vi "디버깅실습(해당 조건부터 하이라이트).vi"() -> ()   [LabVIEW 2020]
panel:
  out "에러 출력":errorcluster
  out "불리언":bool
  out "숫자형":i32
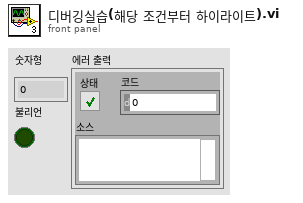
[diagram p1: front panel]
types:
  T1 = enum16{"open", "replace", "create", "open or create", "replace or create", "replace or create with confirmation"}
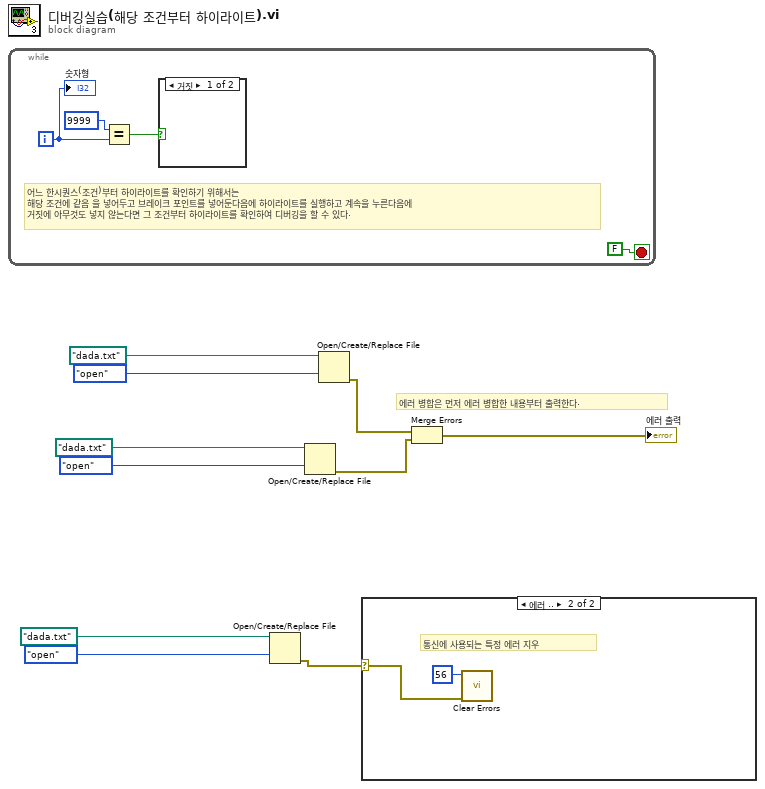
[diagram p0: block diagram]
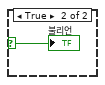
[diagram p3: hidden frame]
diagram:
  # "에러 병합은 먼저 에러 병합한 내용부터 출력한다."
  n1 = while {
    i -> [w12]
    stop <- FALSE stop-if-true
    # "어느 한시퀀스(조건)부터 하이라이트를 확인하기 위해서는\n해당 조건에 같음 을 넣어두고 브레이크 포인트를 넣어둔다음에 하이라이트를 실행하고 계속을 누른다음에\n거짓에 아무것도 넣지 않는다면 그 조건부터 하이라이트를 확인하여 디버깅을 할 수 있다."
    n2 = Equal?(x=9999, y=w12) -> (x = y?=w11:bool)
    n3 = case shown="거짓" w11 {
      selector: w11 -> [_ w15]
      frame False {
      }
      frame True {
        "불리언" <- w15
      }
    }
    "숫자형" <- w12
  }
  n4 = Open/Create/Replace File(file path (use dialog)=path "dada.txt" ("파일 경로(대화 상자 사용)"), operation (0:open)=T1."open" ("동작(0:open)")) -> (error out=w1:errorcluster)  [unwired: 4 in, 2 out]
  n5 = Open/Create/Replace File(file path (use dialog)=path "dada.txt" ("파일 경로(대화 상자 사용)"), operation (0:open)=T1."open" ("동작(0:open)")) -> (error out=w5:errorcluster)  [unwired: 4 in, 2 out]
  n6 = Open/Create/Replace File(file path (use dialog)=path "dada.txt" ("파일 경로(대화 상자 사용)"), operation (0:open)=T1."open" ("동작(0:open)")) -> (error out=w6:errorcluster)  [unwired: 4 in, 2 out]
  n7 = case shown="에러 .." w1 {
    selector: w1 -> [_ w16]
    frame No Error {
    }
    frame Error {
      # "통신에 사용되는 특정 에러 지우"
      n8 = call <vilib>:"Clear Errors.vi"("error in (no error)"=w16, "specific error code to clear (0: all)"=56) -> ()  [unwired: 4 in, 2 out]
    }
  }
  n9 = Merge Errors(w6, w5) -> (→"에러 출력":errorcluster)
